vi "Main_Mesurement_FPGA.vi"() -> ()   [LabVIEW 2018]
uses:
  <vilib>/rvi/Emulation/niFpgaGetClockAttributes.vi
  <vilib>/rvi/Emulation/niFpgaSctlEmulationGetInTimedLoop.vi
  <vilib>/rvi/Emulation/niFpgaEmulationReportErrorSimple.vi
  <vilib>/rvi/eio/common/nirviEmuTemplateMethod_errors.vi
  <vilib>/rvi/interface/RandomDataEmulation/niFpgaRandomDataHandleErrors.vi
  <vilib>/rvi/Emulation/niFpgaCriticalErrorInLSC.vi
  <vilib>/eio/EIONode/EIONode.xnode
  <vilib>/rvi/DataTransferAndStorage/Container/XNode/niFpgaContainer.xnode
  <vilib>/rvi/interface/RandomDataEmulation/nirviRandomDataFpgaReadWriteTemplate.vi
panel:
  in  "Timeout 2":i32
  in  "Timeout":i32=1
  in  "TC Loop rate":u32=2 caption="Count(uSec)"
  in  "STOP 2":bool
  in  "Stop":bool
  in  "Loop Rate (uS)":u32=100
  out "Timeout Counter":u64
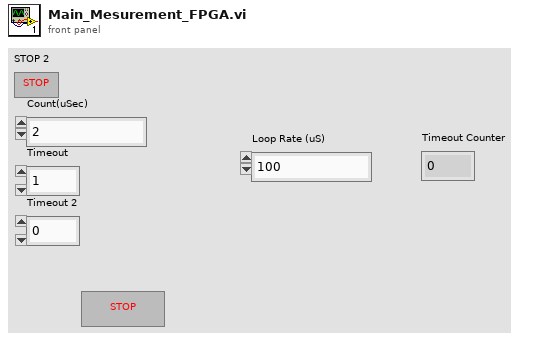
[diagram p1: front panel]
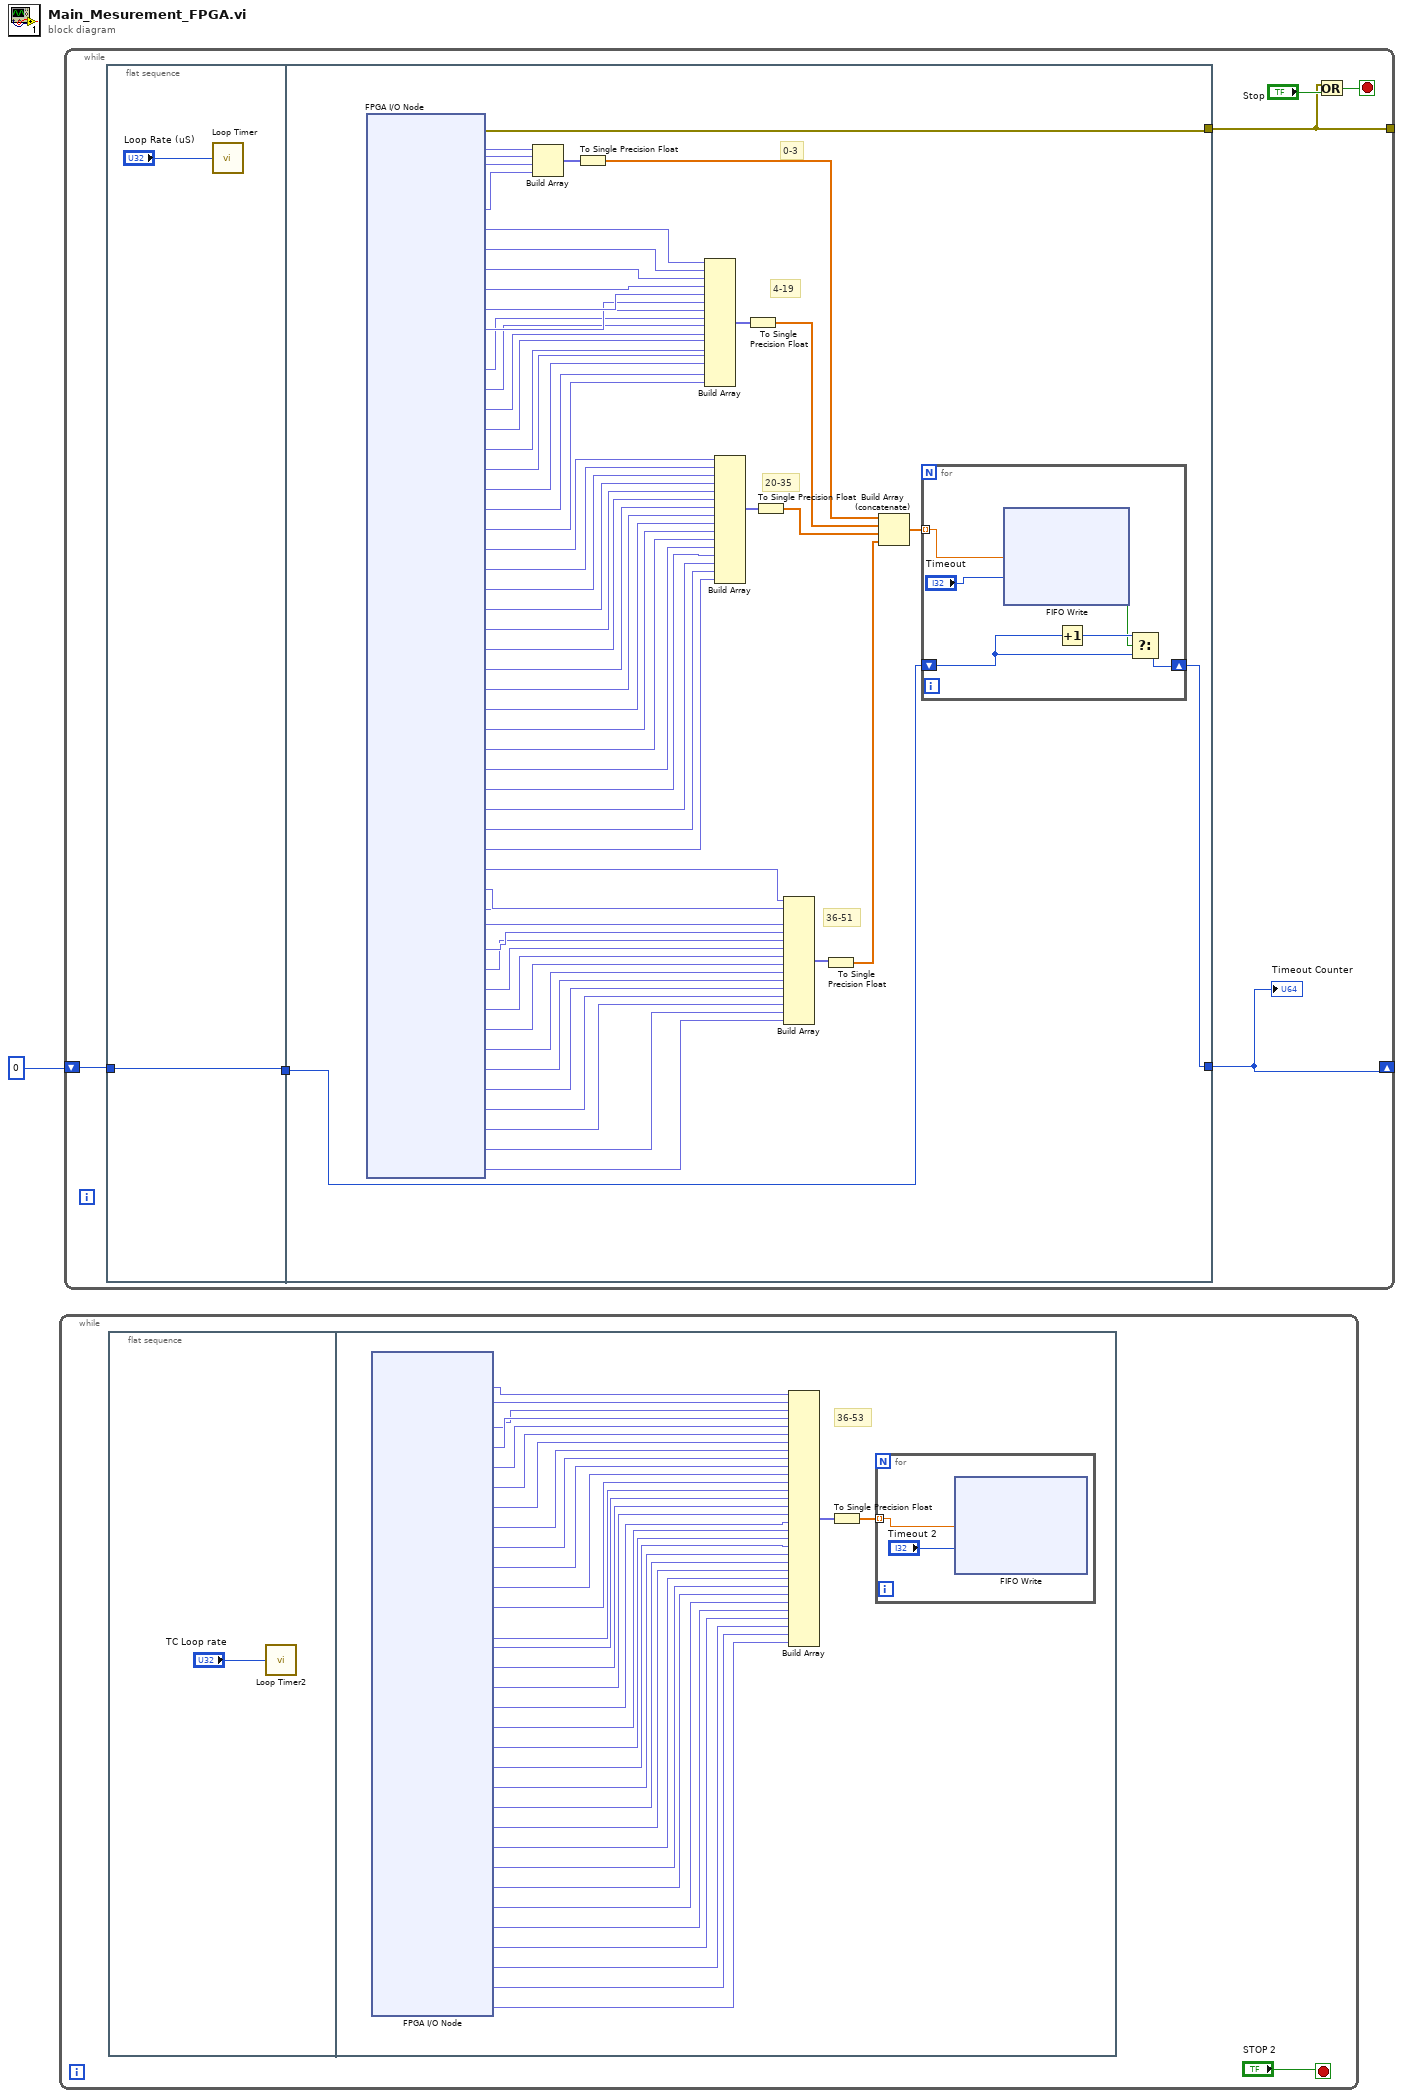
[diagram p0: block diagram]
diagram:
  n1 = while {
    stop <- "STOP 2" stop-if-true
    n2 = flat-sequence {
      frame #0 {
        n3 = call "Loop Timer2"("Count(uSec)"="TC Loop rate") -> ()  [unwired: 1 out]
      }
      frame #1 {
        # "36-53"
        n4 = xnode "FPGA I/O Node"() -> ("Mod7/TC0"=w21:fxp<+/-,24,-2>, "Mod7/TC1"=w22:fxp<+/-,24,-2>, "Mod7/TC2"=w23:fxp<+/-,24,-2>, "Mod7/TC3"=w24:fxp<+/-,24,-2>, "Mod7/TC4"=w25:fxp<+/-,24,-2>, "Mod7/TC5"=w26:fxp<+/-,24,-2>, "Mod7/TC6"=w27:fxp<+/-,24,-2>, "Mod7/TC7"=w28:fxp<+/-,24,-2>, "Mod7/TC8"=w29:fxp<+/-,24,-2>, "Mod7/TC9"=w30:fxp<+/-,24,-2>, "Mod7/TC10"=w31:fxp<+/-,24,-2>, "Mod7/TC11"=w32:fxp<+/-,24,-2>, "Mod7/TC12"=w33:fxp<+/-,24,-2>, "Mod7/TC13"=w34:fxp<+/-,24,-2>, "Mod7/TC14"=w35:fxp<+/-,24,-2>, "Mod7/TC15"=w36:fxp<+/-,24,-2>, "Mod8/TC0"=w19:fxp<+/-,24,-2>, "Mod8/TC1"=w18:fxp<+/-,24,-2>, "Mod8/TC2"=w17:fxp<+/-,24,-2>, "Mod8/TC3"=w16:fxp<+/-,24,-2>, "Mod8/TC4"=w15:fxp<+/-,24,-2>, "Mod8/TC5"=w14:fxp<+/-,24,-2>, "Mod8/TC6"=w13:fxp<+/-,24,-2>, "Mod8/TC7"=w12:fxp<+/-,24,-2>, "Mod8/TC8"=w11:fxp<+/-,24,-2>, "Mod8/TC9"=w10:fxp<+/-,24,-2>, "Mod8/TC10"=w9:fxp<+/-,24,-2>, "Mod8/TC11"=w8:fxp<+/-,24,-2>, "Mod8/TC12"=w7:fxp<+/-,24,-2>, "Mod8/TC13"=w6:fxp<+/-,24,-2>, "Mod8/TC14"=w5:fxp<+/-,24,-2>, "Mod8/TC15"=w4:fxp<+/-,24,-2>)  [unwired: 33 in, 33 out]
        n5 = Build Array(w21, w22, w23, w24, w25, w26, w27, w28, w29, w30, w31, w32, w33, w34, w35, w36, w19, w18, w17, w16, w15, w14, w13, w12, w11, w10, w9, w8, w7, w6, w5, w4) -> (w37:fxp<+/-,24,-2>[])
        n6 = To Single Precision Float(number=w37) -> (single precision float=w20:sgl[])
        n7 = for {
          tunnel: w20 -> [w38] mode=indexing
          n8 = xnode ("FIFO Write")("Element"=w38, "Timeout"="Timeout 2") -> ()  [unwired: 1 in, 2 out]
        }
      }
    }
  }
  n9 = while {
    tunnel: [w43] -> _
    shift-right: [w40] -> _
    shift-left: u64 0 -> [w41]
    stop <- w44 stop-if-true
    n10 = flat-sequence {
      tunnel: [w46] -> w42
      tunnel: w41 -> [w46]
      tunnel: [w111] -> w43
      tunnel: w42 -> [w110]
      tunnel: [w109] -> w40
      frame #0 {
        n11 = call "Loop Timer"("Count(uSec)"="Loop Rate (uS)") -> ()  [unwired: 1 out]
      }
      frame #1 {
        # "36-51"
        # "20-35"
        # "4-19"
        # "0-3"
        n12 = xnode "FPGA I/O Node"() -> ("error out"=w111:errorcluster, "Mod1/CH0"=w92:fxp<+/-,32,-1>, "Mod1/CH1"=w91:fxp<+/-,32,-1>, "Mod1/CH2"=w90:fxp<+/-,32,-1>, "Mod1/CH3"=w89:fxp<+/-,32,-1>, "Mod2/AI0"=w108:fxp<+/-,24,5>, "Mod2/AI1"=w107:fxp<+/-,24,5>, "Mod2/AI2"=w106:fxp<+/-,24,5>, "Mod2/AI3"=w105:fxp<+/-,24,5>, "Mod2/AI4"=w104:fxp<+/-,24,5>, "Mod2/AI5"=w103:fxp<+/-,24,5>, "Mod2/AI6"=w102:fxp<+/-,24,5>, "Mod2/AI7"=w101:fxp<+/-,24,5>, "Mod2/AI8"=w100:fxp<+/-,24,5>, "Mod2/AI9"=w99:fxp<+/-,24,5>, "Mod2/AI10"=w98:fxp<+/-,24,5>, "Mod2/AI11"=w97:fxp<+/-,24,5>, "Mod2/AI12"=w96:fxp<+/-,24,5>, "Mod2/AI13"=w95:fxp<+/-,24,5>, "Mod2/AI14"=w94:fxp<+/-,24,5>, "Mod2/AI15"=w93:fxp<+/-,24,5>, "Mod4/AI0"=w84:fxp<+/-,24,-4>, "Mod4/AI1"=w83:fxp<+/-,24,-4>, "Mod4/AI2"=w82:fxp<+/-,24,-4>, "Mod4/AI3"=w81:fxp<+/-,24,-4>, "Mod4/AI4"=w80:fxp<+/-,24,-4>, "Mod4/AI5"=w79:fxp<+/-,24,-4>, "Mod4/AI6"=w78:fxp<+/-,24,-4>, "Mod4/AI7"=w77:fxp<+/-,24,-4>, "Mod4/AI8"=w76:fxp<+/-,24,-4>, "Mod4/AI9"=w75:fxp<+/-,24,-4>, "Mod4/AI10"=w74:fxp<+/-,24,-4>, "Mod4/AI11"=w73:fxp<+/-,24,-4>, "Mod4/AI12"=w72:fxp<+/-,24,-4>, "Mod4/AI13"=w68:fxp<+/-,24,-4>, "Mod4/AI14"=w67:fxp<+/-,24,-4>, "Mod4/AI15"=w66:fxp<+/-,24,-4>, "Mod3/AI0"=w65:fxp<+/-,24,5>, "Mod3/AI1"=w64:fxp<+/-,24,5>, "Mod3/AI2"=w63:fxp<+/-,24,5>, "Mod3/AI3"=w62:fxp<+/-,24,5>, "Mod3/AI4"=w61:fxp<+/-,24,5>, "Mod3/AI5"=w60:fxp<+/-,24,5>, "Mod3/AI6"=w59:fxp<+/-,24,5>, "Mod3/AI7"=w58:fxp<+/-,24,5>, "Mod3/AI8"=w57:fxp<+/-,24,5>, "Mod3/AI9"=w56:fxp<+/-,24,5>, "Mod3/AI10"=w55:fxp<+/-,24,5>, "Mod3/AI11"=w54:fxp<+/-,24,5>, "Mod3/AI12"=w53:fxp<+/-,24,5>, "Mod3/AI13"=w52:fxp<+/-,24,5>, "Mod3/AI14"=w49:fxp<+/-,24,5>, "Mod3/AI15"=w48:fxp<+/-,24,5>)  [unwired: 53 in, 52 out]
        n13 = Build Array(w92, w91, w90, w89) -> (w88:fxp<+/-,32,-1>[])
        n14 = To Single Precision Float(number=w88) -> (single precision float=w87:sgl[])
        n15 = Build Array(w108, w107, w106, w105, w104, w103, w102, w101, w100, w99, w98, w97, w96, w95, w94, w93) -> (w86:fxp<+/-,24,5>[])
        n16 = Build Array(w84, w83, w82, w81, w80, w79, w78, w77, w76, w75, w74, w73, w72, w68, w67, w66) -> (w71:fxp<+/-,24,-4>[])
        n17 = To Single Precision Float(number=w86) -> (single precision float=w85:sgl[])
        n18 = To Single Precision Float(number=w71) -> (single precision float=w70:sgl[])
        n19 = Build Array(w65, w64, w63, w62, w61, w60, w59, w58, w57, w56, w55, w54, w53, w52, w49, w48) -> (w51:fxp<+/-,24,5>[])
        n20 = To Single Precision Float(number=w51) -> (single precision float=w50:sgl[])
        n21 = Build Array (concatenate)(w87, w85, w70, w50) -> (w69:sgl[])
        n22 = for {
          shift-right: [w115] -> w109
          shift-left: w110 -> [w117]
          tunnel: w69 -> [w112] mode=indexing
          n23 = xnode ("FIFO Write")("Element"=w112, "Timeout"="Timeout") -> ("Timed Out?"=w113:bool)  [unwired: 1 in, 1 out]
          n24 = Increment(x=w117) -> (x+1=w116:u64)
          n25 = Select(t=w116, s=w113, f=w117) -> (s? t:f=w115:u64)
        }
      }
    }
    n26 = Or(x=w43, y="Stop") -> (x .or. y?=w44:bool)
    "Timeout Counter" <- w40
  }
